vi "Description Panel.vi"(8 "error in (no error)":errorcluster, 9 "Description":string, 10 "Description Title":string) -> (0 "error out":errorcluster, 3 "Description Panel out":refnum<class "Description Panel.lvclass">)   [LabVIEW 2017, in "2. Basic Panel Actors.lvlib" / "Description Panel.lvclass"]
doc: "Initializes a new Description panel actor.\n----\nCopyright: MGI 2017\nAuthor: Derek Trepanier"
uses:
  Description Panel.lvclass
  Description Panel.lvclass/Description Panel.ctl
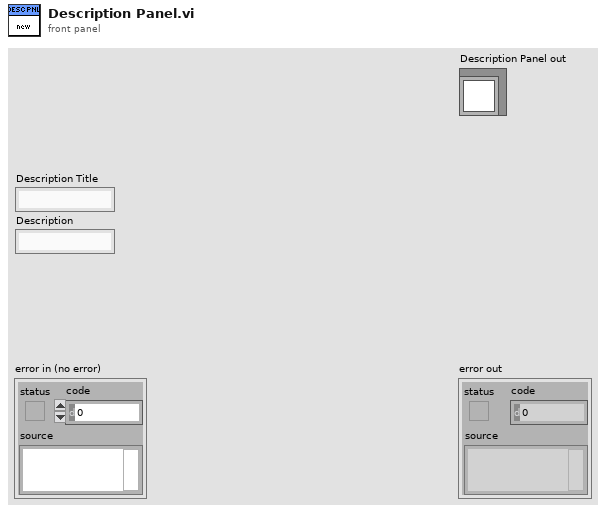
[diagram p1: front panel]
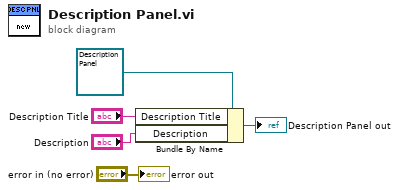
[diagram p0: block diagram]
diagram:
  n1 = Bundle By Name(cluster=refnum<class "Description Panel.lvclass"> refnum ("Description Panel in"), "Description Title"="Description Title", "Description"="Description") -> (→"Description Panel out":refnum<class "Description Panel.lvclass">)
  "error out" <- "error in (no error)"
